vi "Begin.vi"(11 "Image Size":T1=enum."160x120") -> (0 "error out":errorcluster)   [LabVIEW 2011]
doc: "Called before other user functions, this VI is expected to open initial I/O refnums, load in file data, and do all program initialization. Notice that the <B>error out</B> terminal is simply used for data flow. Wiring it to other structures or subVIs ensures that this VI runs first."
uses:
  <vilib>/Rock Robotics/WPI/Camera/WPI_CameraImageSize.ctl
  <vilib>/Rock Robotics/SystemInterfaces/DIO/FPGA_DIOPWMChannel.ctl
  <vilib>/Rock Robotics/WPI/Joystick/WPI_JoystickDeviceEnum.ctl
  <vilib>/Rock Robotics/WPI/Camera/WPI_CameraWhite Balance Values.ctl
  <vilib>/Rock Robotics/WPI/Camera/WPI_CameraExposure Values.ctl
  <vilib>/Rock Robotics/WPI/Camera/WPI_CameraFrameRate.ctl
  <vilib>/Rock Robotics/WPI/RobotDrive/WPI_RobotDriveOpen2MotorWithJaguar.vi
  <vilib>/Rock Robotics/WPI/MotorControl/WPI_MotorControlOpen Jaguar.vi
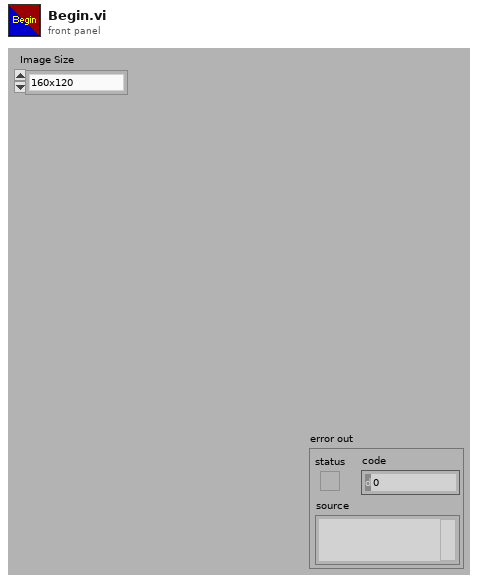
[diagram p1: front panel]
types:
  T1 = typedef "WPI_CameraImageSize.ctl" = enum16{"640x480", "320x240", "160x120"}
  T2 = typedef "FPGA_DIOPWMChannel.ctl" = enum8{"PWM 1", "PWM 2", "PWM 3", "PWM 4", "PWM 5", "PWM 6", "PWM 7", "PWM 8", "PWM 9", "PWM 10", "Invalid"}
  T3 = typedef "WPI_JoystickDeviceEnum.ctl" = enum16{"USB 1", "USB 2", "USB 3", "USB 4", "Kinect 1", "Kinect 2"}
  T4 = typedef "WPI_CameraFrameRate.ctl" = u32
  T5 = typedef "WPI_CameraExposure Values.ctl" = enum16{"Auto", "Flicker-free 50 Hz", "Flicker-free 60 Hz", "Hold current"}
  T6 = typedef "WPI_CameraWhite Balance Values.ctl" = enum16{"Auto", "Fixed indoor", "Fixed outdoor 1", "Fixed outdoor 2", "Fixed fluorescent 1", "Fixed fluorescent 2", "Hold current"}
  T7 = typedef "WPI_JoystickDevRef.ctl" = cluster{"Device":T3}
  T8 = typedef "WPI_MotorControlDeviceRef.ctl" = cluster{"DeviceStatus":errorcluster, "Type":enum16{"PWM", "CAN"}, "PWM":cluster{"Digital Module":T9, "PWM Channel":T2, "DeadBand":T10}, "CAN":cluster{"Device Number":u8, "Control Mode":T11, "Semaphore":T12, "Max Vout":dbl}, "Invert":bool, "TransformRef":T13, "InvTransformRef":T13}
  T9 = typedef "FPGA_TypedefDigitalModule.ctl" = enum16{"Digital Module 1", "Digital Module 2"}
  T10 = typedef "WPI_PWMDeadband.ctl" = cluster{"Name":string, "maxPositivePwm":i32, "minPositivePwm":i32, "centerPwm":i32, "maxNegativePwm":i32, "minNegativePwm":i32, "angularRange":u16}
  T11 = typedef "WPI_CANJaguar_ControlMode.ctl" = enum8{"Percent VBus", "Current", "Speed", "Position", "Voltage"}
  T12 = typedef "Semaphore RefNum" = refnum<k1>
  T13 = typedef "WPI_PWMTransform_ConPane.ctl" = refnum<vi>
  T14 = typedef "WPI_RobotDriveDevRef.ctl" = cluster{"DevStatus":errorcluster, "Motors[]":T8[], "Square Inputs":bool, "Max Output":dbl, "Isochronous":bool}
  T15 = typedef "WPI_CameraDevRef.ctl" = cluster{"Camera Address":string, "CameraStatus":errorcluster, "Acquire Image Notifier":refnum<notifier>}
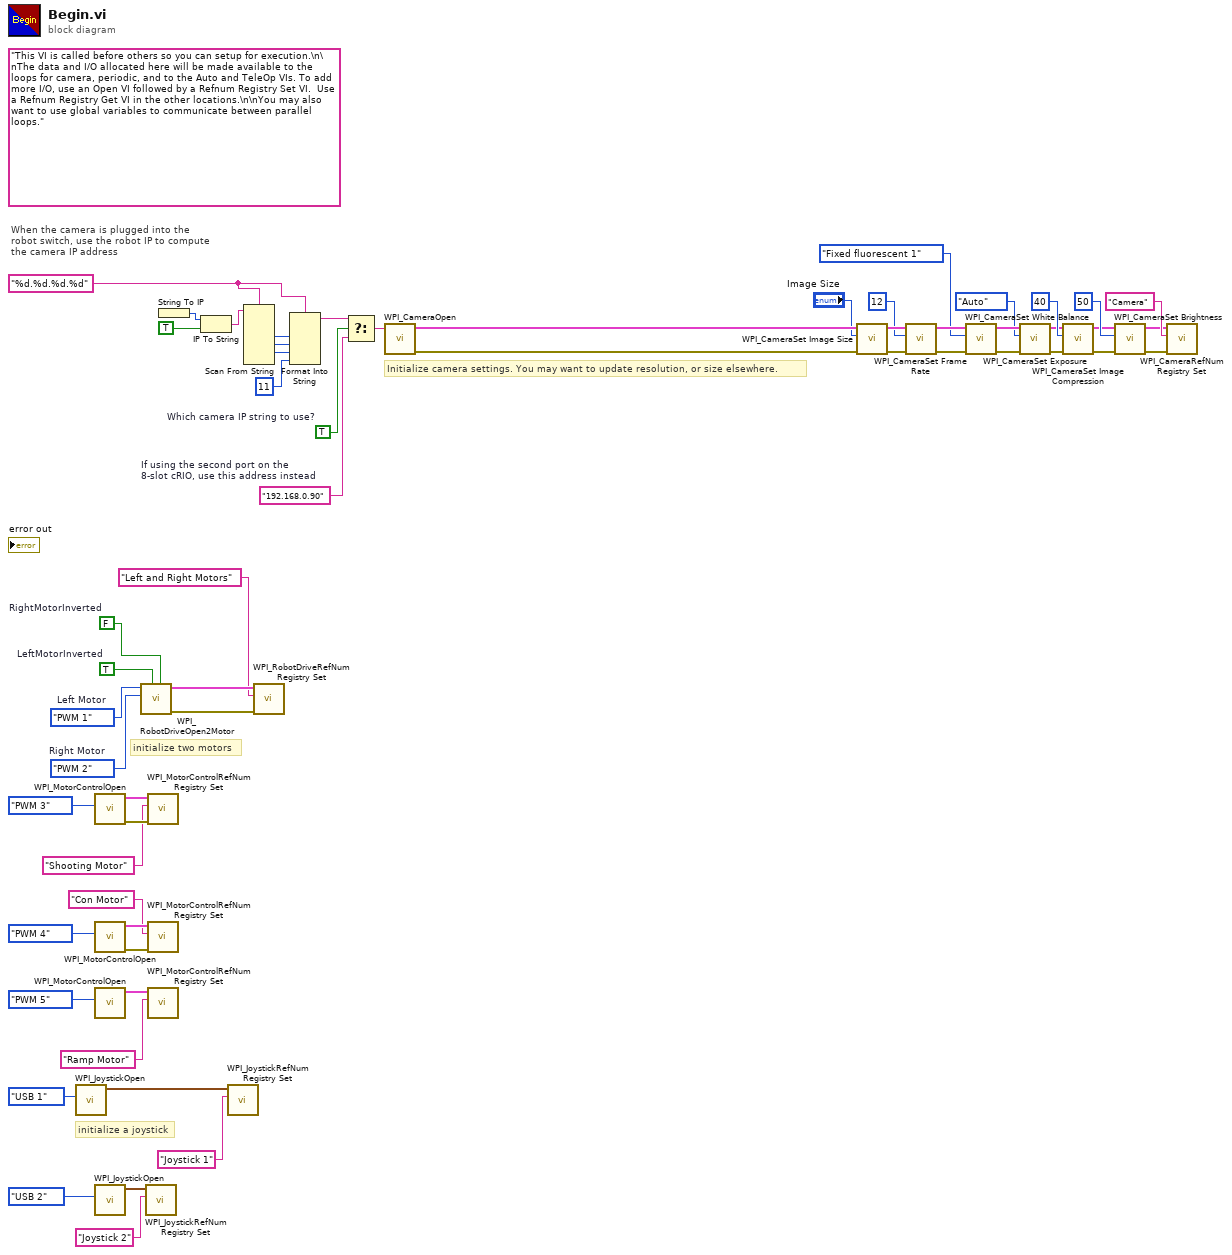
[diagram p0: block diagram]
diagram:
  w15 = TRUE  # Which camera IP string to use?
  w19 = "%d.%d.%d.%d" ("format string")
  (unwired) "This VI is called before others so you can setup for execution.\n\nThe data and I/O allocated here will be made available to the loops for camera, periodic, and to the Auto and TeleOp VIs. To add more I/O, use an Open VI followed by a Refnum Registry Set VI.  Use a Refnum Registry Get VI in the other locations.\n\nYou may also want to use global variables to communicate between parallel loops."
  w31 = FPGA_DIOPWMChannel."PWM 2"  # Right Motor
  w32 = FPGA_DIOPWMChannel."PWM 1"  # Left Motor
  w16 = "192.168.0.90"  # If using the second port on the 8-slot cRIO, use this address instead
  w56 = TRUE  # LeftMotorInverted
  w57 = FALSE  # RightMotorInverted
  # "When the camera is plugged into the\nrobot switch, use the robot IP to compute\nthe camera IP address"
  # "initialize a joystick"
  # "initialize two motors"
  # "Initialize camera settings. You may want to update resolution, or size elsewhere."
  n1 = call <vilib>:"WPI_JoystickOpen.vi"("JoystickDevice"=WPI_JoystickDeviceEnum."USB 1") -> ("JoystickDevRef"=w52:T7)  [unwired: 10 out]
  n2 = call-poly <vilib>:"WPI_MotorControlOpen.vi"("PWM Channel"=FPGA_DIOPWMChannel."PWM 3") -> ("error out"=w10:errorcluster, "MotorControlDeviceRef"=w11:T8)  [unwired: 9 in]
  n3 = call-poly <vilib>:"WPI_MotorControlOpen.vi"("PWM Channel"=FPGA_DIOPWMChannel."PWM 4") -> ("error out"=w6:errorcluster, "MotorControlDeviceRef"=w7:T8)  [unwired: 9 in]
  n4 = call-poly <vilib>:"WPI_MotorControlOpen.vi"("PWM Channel"=FPGA_DIOPWMChannel."PWM 5") -> ("MotorControlDeviceRef"=w1:T8)  [unwired: 9 in, 1 out]
  n5 = call <vilib>:"WPI_JoystickOpen.vi"("JoystickDevice"=WPI_JoystickDeviceEnum."USB 2") -> ("JoystickDevRef"=w14:T7)  [unwired: 10 out]
  n6 = call-poly <vilib>:"WPI_RobotDriveOpen2Motor.vi"("Right Motor Inverted"=w57, "Left Motor Inverted"=w56, "Right Motor"=w31, "Left Motor"=w32) -> ("error out"=w50:errorcluster, "RobotDriveDevRef"=w54:T14)  [unwired: 1 in, 5 out]
  n7 = call <vilib>:"WPI_JoystickRefNum Registry Set.vi"("refnum name"="Joystick 2", "JoystickDevRef"=w14) -> ()  [unwired: 1 in, 9 out]
  n8 = call <vilib>:"WPI_MotorControlRefNum Registry Set.vi"("error in (no error)"=w10, "refnum name"="Shooting Motor", "MotorControlDevRef"=w11) -> ()  [unwired: 7 in, 2 out]
  n9 = call <vilib>:"WPI_MotorControlRefNum Registry Set.vi"("error in (no error)"=w6, "refnum name"="Con Motor", "MotorControlDevRef"=w7) -> ()  [unwired: 7 in, 2 out]
  n10 = call <vilib>:"WPI_MotorControlRefNum Registry Set.vi"("refnum name"="Ramp Motor", "MotorControlDevRef"=w1) -> ()  [unwired: 8 in, 2 out]
  n11 = String To IP() -> (0:w26:u32)  [unwired: 1 in]
  n12 = IP To String(1:TRUE ("dot notation? (F)"), 2:w26) -> (0:w24:string)
  n13 = call <vilib>:"WPI_JoystickRefNum Registry Set.vi"("refnum name"="Joystick 1", "JoystickDevRef"=w52) -> ()  [unwired: 1 in, 9 out]
  n14 = Scan From String(format string=w19, input string=w24) -> (output 1=w23:i32, output 2=w22:i32, output 3=w21:i32)  [unwired: 7 in, 3 out]
  n15 = call <vilib>:"WPI_RobotDriveRefNum Registry Set.vi"("error in (no error)"=w50, "refnum name"="Left and Right Motors", "RobotDriveDevRef"=w54) -> ()  [unwired: 9 out]
  n16 = Format Into String(format string=w19, w23, w22, w21, 11 ("Compression")) -> (resulting string=w17:string)  [unwired: 2 in, 1 out]
  n17 = Select(t=w17, s=w15, f=w16) -> (s? t:f=w18:string)
  n18 = call <vilib>:"WPI_CameraOpen.vi"("Camera Address"=w18) -> ("error out"=w41:errorcluster, "CameraDevRef"=w42:T15)  [unwired: 1 in, 8 out]
  n19 = call <vilib>:"WPI_CameraSet Image Size.vi"("error in (no error)"=w41, "Image Size"="Image Size", "CameraDevRef"=w42) -> ("error out"=w40:errorcluster, "CameraDevRef Out"=w43:T15)  [unwired: 7 out]
  n20 = call <vilib>:"WPI_CameraSet Frame Rate.vi"("error in (no error)"=w40, "Frame Rate (fps)"=T4 12, "CameraDevRef"=w43) -> ("error out"=w39:errorcluster, "CameraDevRef Out"=w45:T15)  [unwired: 7 out]
  n21 = call <vilib>:"WPI_CameraSet White Balance.vi"("error in (no error)"=w39, "White Balance"=WPI_CameraWhite_Balance_Values."Fixed fluorescent 1", "CameraDevRef"=w45) -> ("error out"=w38:errorcluster, "CameraDevRef Out"=w44:T15)  [unwired: 7 out]
  n22 = call <vilib>:"WPI_CameraSet Exposure.vi"("error in (no error)"=w38, "Exposure"=WPI_CameraExposure_Values."Auto", "CameraDevRef"=w44) -> ("error out"=w37:errorcluster, "CameraDevRef Out"=w47:T15)  [unwired: 7 out]
  n23 = call <vilib>:"WPI_CameraSet Image Compression.vi"("error in (no error)"=w37, "Compression"=40, "CameraDevRef"=w47) -> ("error out"=w36:errorcluster, "CameraDevRef Out"=w46:T15)  [unwired: 7 out]
  n24 = call <vilib>:"WPI_CameraSet Brightness.vi"("error in (no error)"=w36, "Brightness"=50, "CameraDevRef"=w46) -> ("error out"=w34:errorcluster, "CameraDevRef Out"=w35:T15)  [unwired: 7 out]
  n25 = call <vilib>:"WPI_CameraRefNum Registry Set.vi"("error in (no error)"=w34, "refnum name"="Camera", "CameraDevRef"=w35) -> ()  [unwired: 9 out]
